vi "getPath.vi"(11 "Numeric":i32=2) -> (1 "cam2":path=path "cam2", 2 "cam1":path, 3 "cam0":path, 4 "cam3":path)   [LabVIEW 2011]
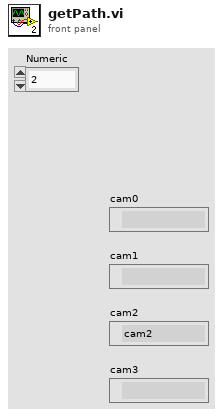
[diagram p1: front panel]
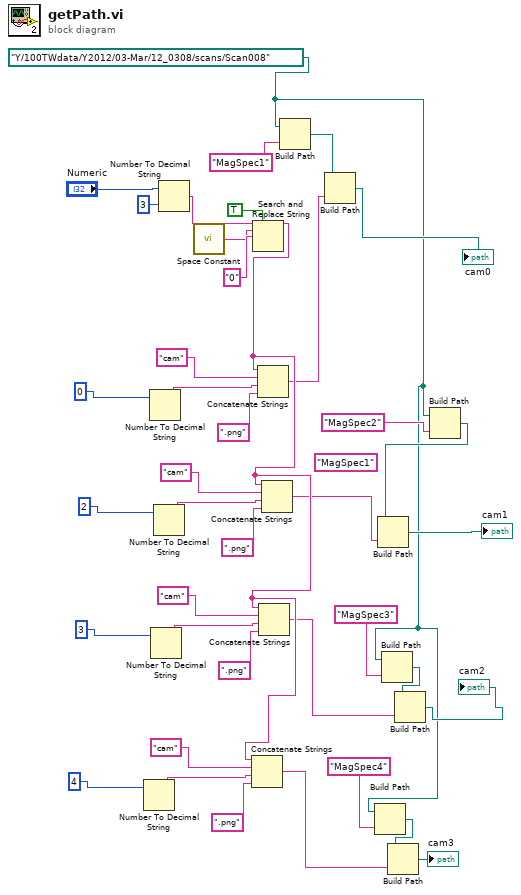
[diagram p0: block diagram]
diagram:
  (unwired) "MagSpec1" ("name or relative path")
  w1 = path "Y:/100TWdata/Y2012/03-Mar/12_0308/scans/Scan008" ("image 2")
  n1 = Number To Decimal String(number=4) -> (decimal integer string=w36:string)  [unwired: 1 in]
  n2 = Number To Decimal String(number=0) -> (decimal integer string=w10:string)  [unwired: 1 in]
  n3 = Number To Decimal String(number=3) -> (decimal integer string=w26:string)  [unwired: 1 in]
  n4 = Number To Decimal String(number=2) -> (decimal integer string=w15:string)  [unwired: 1 in]
  n5 = Number To Decimal String(number="Numeric", width (-)=i16 3) -> (decimal integer string=w4:string)
  n6 = call "Space Constant.vi"() -> ("String"=w5:string)
  n7 = Search and Replace String(replace all?=TRUE ("replace all? (F)"), input string=w4, search string=w5, replace string="0") -> (result string=w39:string)  [unwired: 4 in, 3 out]
  n8 = Concatenate Strings(w39, "cam", w36, ".png" ("string")) -> (w33:string)
  n9 = Concatenate Strings(w39, "cam", w10, ".png" ("string")) -> (w12:string)
  n10 = Concatenate Strings(w39, "cam", w26, ".png" ("string")) -> (w29:string)
  n11 = Concatenate Strings(w39, "cam", w15, ".png" ("string")) -> (w20:string)
  n12 = Build Path(base path=w1, name or relative path="MagSpec1") -> (appended path=w19:path)
  n13 = Build Path(base path=w19, name or relative path=w12) -> (appended path=→"cam0":path)
  n14 = Build Path(base path=w1, name or relative path="MagSpec4") -> (appended path=w32:path)
  n15 = Build Path(base path=w1, name or relative path="MagSpec3") -> (appended path=w30:path)
  n16 = Build Path(base path=w32, name or relative path=w33) -> (appended path=→"cam3":path)
  n17 = Build Path(base path=w30, name or relative path=w29) -> (appended path=→"cam2":path)
  n18 = Build Path(base path=w1, name or relative path="MagSpec2") -> (appended path=w22:path)
  n19 = Build Path(base path=w22, name or relative path=w20) -> (appended path=→"cam1":path)
